vi "Test Get Map Default Values.vi"() -> ()   [LabVIEW 2020]
uses:
  d02e6255-45fc-4346-87ee-8890abef741f.vi
  <vilib>/addons/_JKI Toolkits/Caraya/classes/Assert/Assert Equal Value and Type_Variant.vi
  <vilib>/addons/_JKI Toolkits/Caraya/classes/Test/Test.lvclass
  <vilib>/addons/_JKI Toolkits/Caraya/classes/Assert/Assert.lvclass
panel:
  out "error out":errorcluster
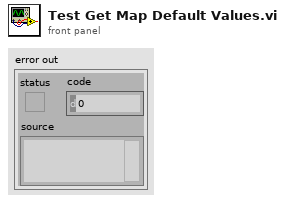
[diagram p1: front panel]
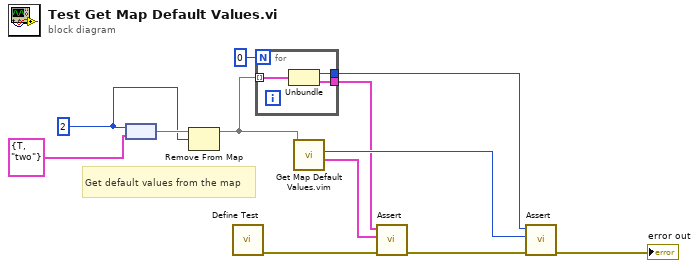
[diagram p0: block diagram]
diagram:
  w5 = 2 ("Name")
  # "Get default values from the map"
  n1 = node(w5, cluster{"bool":bool, "string":string} {"bool"=TRUE, "string"="two"} ("value")) -> (w6:map{i32, cluster{"bool":bool, "string":string}})
  n2 = Remove From Map(10:w5, 11:w6) -> (3:w4:map{i32, cluster{"bool":bool, "string":string}})  [unwired: 2 out]
  n3 = call <vilib>:"Define Test.vi"() -> ("error out"=w9:errorcluster)  [unwired: 11 in]
  n4 = for {
    N: 0 -> [_]
    tunnel: w4 -> [w13] mode=indexing
    tunnel: [w15] -> w3
    tunnel: [w14] -> w2
    n5 = Unbundle(w13) -> ("Name"=w15:i32, "value"=w14:cluster{"bool":bool, "string":string})
  }
  n6 = call "Get Map Default Values.vim"("map"=w4) -> ("value"=w10:cluster{"bool":bool, "string":string}, "key"=w11:i32)  [unwired: 9 in]
  n7 = call-poly <vilib>:"Assert.vi"("error in (no error)"=w9, "Y"=w10, "X"=w2) -> ("error out"=w8:errorcluster)  [unwired: 8 in]
  n8 = call-poly <vilib>:"Assert.vi"("error in (no error)"=w8, "Y"=w11, "X"=w3) -> ("error out"=→"error out":errorcluster)  [unwired: 8 in]
